vi "array - generate range V3.vi"(0 "win":T1={"cen (Hz)"=32000.0, "win (Hz)"=1000.0, "left (Hz)"=61142.4563753074, "right (Hz)"=1277846.8491336836}, 1 "scan type":T2, 11 "df":dbl, 12 "N":i32=-1) -> (8 "Array":dbl[](array[numeric]), 15 "df out":dbl)   [LabVIEW 2018]
uses:
  freq scan type.ctl
  show-win- control.ctl
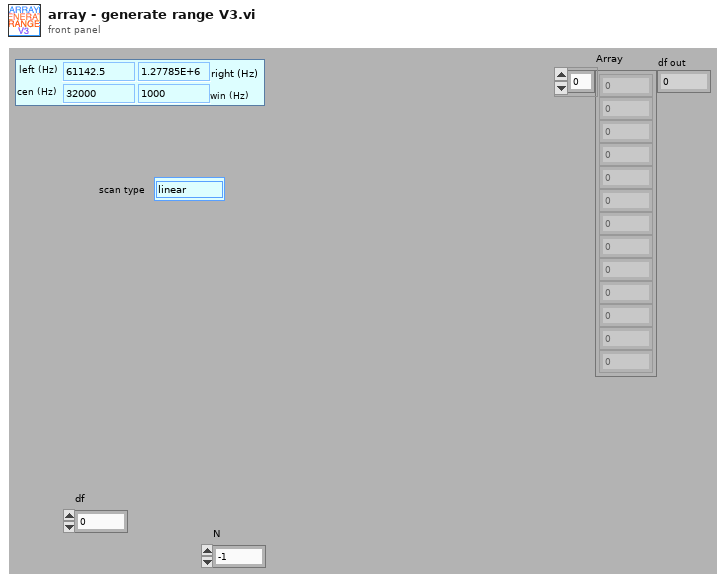
[diagram p1: front panel]
types:
  T1 = typedef "show-win- control.ctl" = cluster{"cen (Hz)":dbl, "win (Hz)":dbl, "left (Hz)":dbl, "right (Hz)":dbl}
  T2 = typedef "freq scan type.ctl" = enum16{"linear", "arctan"}
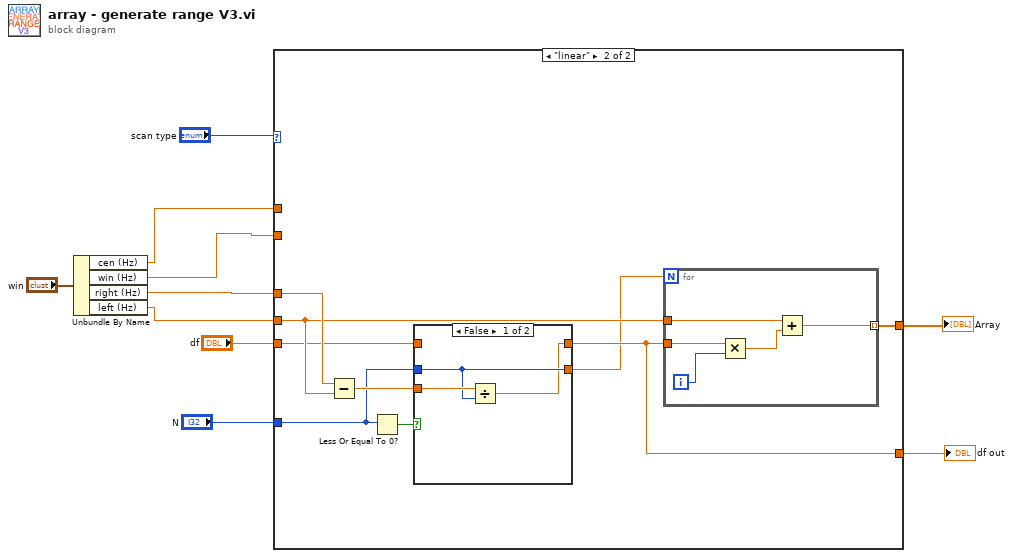
[diagram p0: block diagram]
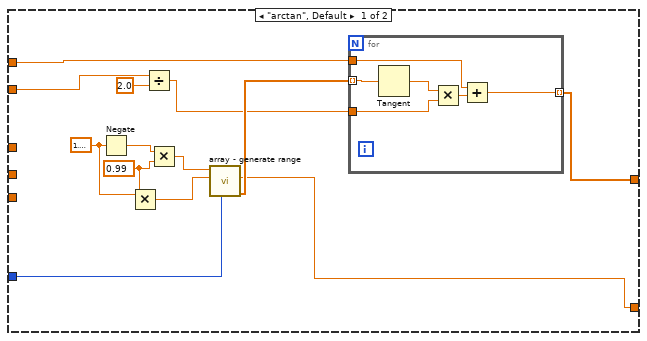
[diagram p2: hidden frame]
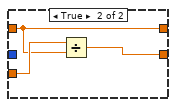
[diagram p3: hidden frame]
diagram:
  n1 = Unbundle By Name("win") -> ("cen (Hz)"=w4:dbl, "win (Hz)"=w3:dbl, "right (Hz)"=w2:dbl, "left (Hz)"=w1:dbl)
  n2 = case shown="\"linear\"" "scan type" {
    tunnel: w2 -> [_ w38]
    tunnel: w1 -> [_ w37]
    tunnel: [w12 w36] -> w10
    tunnel: [w11 w34] -> w9
    tunnel: "df" -> [_ w33]
    tunnel: "N" -> [w13 w30]
    tunnel: w4 -> [w15 _]
    tunnel: w3 -> [w14 _]
    frame "arctan", Default {
      w21 = 0.99
      w22 = 1.5707963267948966
      n3 = Negate(x=w22) -> (-x=w23:dbl)
      n4 = Multiply(x=w22, y=w21) -> (x*y=w19:dbl)
      n5 = Divide(x=w14, y=2.0) -> (x/y=w16:dbl)
      n6 = Multiply(x=w23, y=w21) -> (x*y=w20:dbl)
      n7 = call "array - generate range.vi"("N"=w13, "freq max"=w19, "freq min"=w20) -> ("Array"=w18:dbl[], "df out"=w11:dbl)  [unwired: 7 in]
      n8 = for {
        tunnel: [w29] -> w12 mode=indexing
        tunnel: w18 -> [w27] mode=indexing
        tunnel: w15 -> [w28]
        tunnel: w16 -> [w26]
        n9 = Tangent(1:w27) -> (0:w25:dbl)
        n10 = Multiply(x=w25, y=w26) -> (x*y=w24:dbl)
        n11 = Add(x=w28, y=w24) -> (x+y=w29:dbl)
      }
    }
    frame "linear" {
      n12 = Subtract(x=w38, y=w37) -> (x-y=w32:dbl)
      n13 = Less Or Equal To 0?(x=w30) -> (x <= 0?=w35:bool)
      n14 = case shown="False" w35 {
        tunnel: [w39 w43] -> w34
        tunnel: w33 -> [_ w43]
        tunnel: w32 -> [w41 w44]
        tunnel: [w40 w42] -> w31
        tunnel: w30 -> [w40 _]
        frame False {
          n15 = Divide(x=w41, y=w40) -> (x/y=w39:dbl)
        }
        frame True {
          n16 = Divide(x=w44, y=w43) -> (x/y=w42:dbl)
        }
      }
      n17 = for {
        N: w31 -> [_]
        tunnel: w34 -> [w48]
        tunnel: w37 -> [w46]
        tunnel: [w45] -> w36 mode=indexing
        i -> [w49]
        n18 = Multiply(x=w48, y=w49) -> (x*y=w47:dbl)
        n19 = Add(x=w46, y=w47) -> (x+y=w45:dbl)
      }
    }
  }
  "Array" <- w10
  "df out" <- w9
